vi "PI_Controller.vi"() -> ()   [LabVIEW 2013]
panel:
  out "Input Voltage":dbl
  in  "Coldfinger\nTemperature (K)":dbl=77.0
  in  "Proportional":dbl=3.0
  in  "Integral":dbl
  in  "Heater Current":u16(ring) items=["Low", "Medium", "High"]
  out "Waveform Chart":dbl(graph)
  out "Percentage \nHeater \nOutput":dbl(knob) scale=0.0..100.0
  in  "?":bool
  out "Temperature (K)":dbl
  in  "dt (s)":dbl=0.5
  in  "Temperature \nSetpoint (K)":dbl=100.0
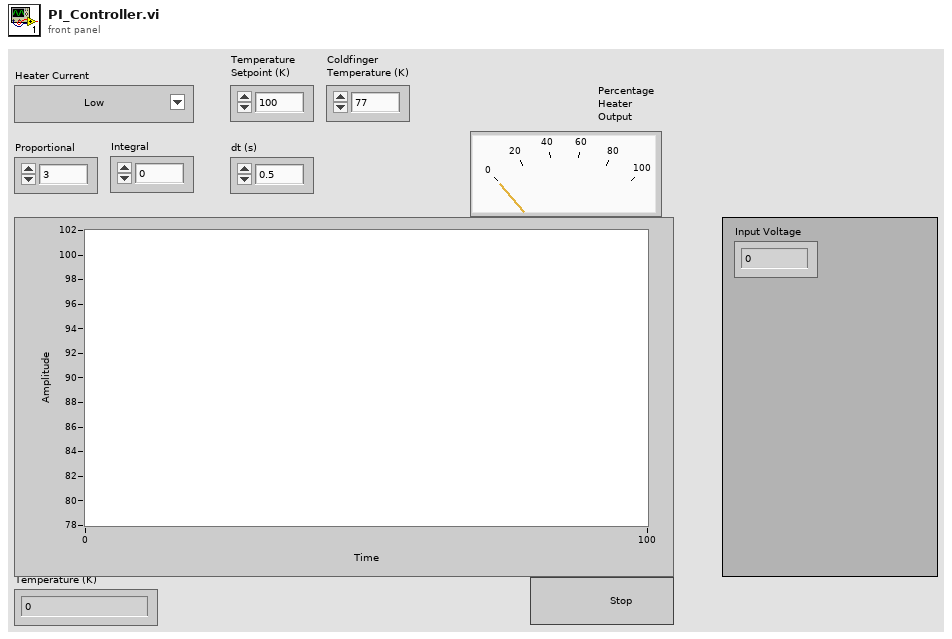
[diagram p1: front panel]
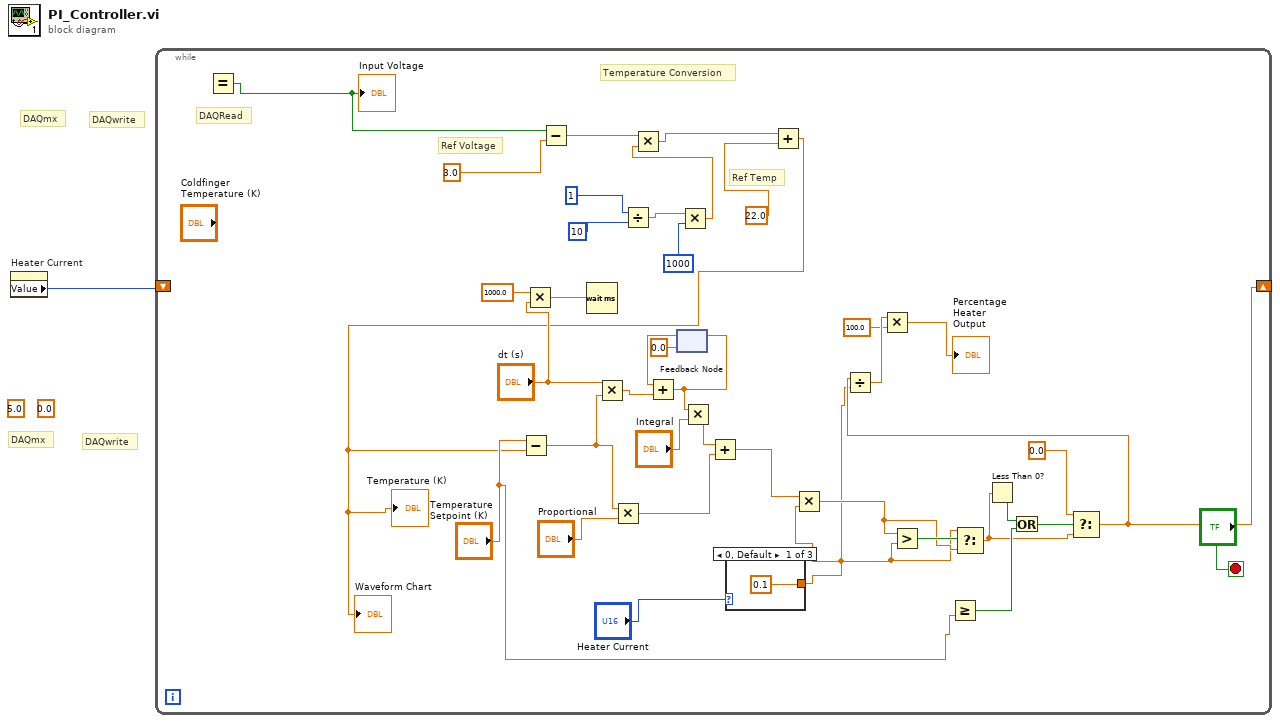
[diagram p0: block diagram]
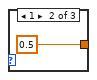
[diagram p2: hidden frame]
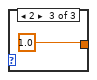
[diagram p3: hidden frame]
diagram:
  (unwired) 0.0
  (unwired) 5.0
  # "DAQwrite"
  # "DAQmx"
  # "DAQwrite"
  # "DAQmx"
  n1 = property on="Heater Current" class="Ring (strict)"() -> ("Value"=w1:u16)  [unwired: 2 in, 2 out]
  n2 = while {
    shift-right: [w17] -> _
    shift-left: w1 -> [_]
    stop <- "?" stop-if-true
    # "Ref Temp"
    # "Ref Voltage"
    # "Temperature Conversion"
    # "DAQRead"
    n3 = Equal?() -> (x = y?=w12:bool)  [unwired: 2 in]
    "Input Voltage" <- w12
    n4 = Multiply(x=sgl 1000.0, y="dt (s)") -> (x*y=w18:dbl)
    n5 = Subtract(x=w12, y=3.0) -> (x-y=w10:dbl)
    n6 = Wait (ms)(milliseconds to wait=w18) -> ()  [unwired: 1 out]
    n7 = Divide(x=1, y=10) -> (x/y=w7:dbl)
    n8 = feedback #1(0.0) -> (w36:dbl)
    n9 = Multiply(x=w7, y=1000) -> (x*y=w5:dbl)
    n10 = Multiply(x=w10, y=w5) -> (x*y=w4:dbl)
    n11 = case shown="0, Default" "Heater Current" {
      tunnel: [0.1 0.5 1.0] -> w16
      frame 0, Default {
      }
      frame 1 {
      }
      frame 2 {
      }
    }
    n12 = Add(x=w4, y=22.0) -> (x+y=w2:dbl)
    "Temperature (K)" <- w2
    "Waveform Chart" <- w2
    n13 = Subtract(x="Temperature \nSetpoint (K)", y=w2) -> (x-y=w38:dbl)
    n14 = Multiply(x="dt (s)", y=w38) -> (x*y=w37:dbl)
    n15 = Multiply(x=w38, y="Proportional") -> (x*y=w32:dbl)
    n16 = Add(x=w36, y=w37) -> (x+y=w34:dbl)
    n17 = feedback-in #1(w34) -> ()
    n18 = Multiply(x=w34, y="Integral") -> (x*y=w31:dbl)
    n19 = Add(x=w31, y=w32) -> (x+y=w30:dbl)
    n20 = Multiply(x=w30, y=w16) -> (x*y=w27:dbl)
    n21 = Greater?(x=w27, y=w16) -> (0:w28:bool)
    n22 = Greater Or Equal?(y="Temperature \nSetpoint (K)") -> (x >= y?=w25:bool)  [unwired: 1 in]
    n23 = Select(t=w16, s=w28, f=w27) -> (s? t:f=w21:dbl)
    n24 = Less Than 0?(x=w21) -> (x < 0?=w26:bool)
    n25 = Or(x=w26, y=w25) -> (x .or. y?=w23:bool)
    n26 = Select(t=0.0, s=w23, f=w21) -> (s? t:f=w17:dbl)
    n27 = Divide(x=w17, y=w16) -> (x/y=w15:dbl)
    n28 = Multiply(x=w15, y=100.0) -> (x*y=→"Percentage \nHeater \nOutput":dbl)
  }
